vi "项名.vi"(8 "error in (no error)":errorcluster caption="错误输入（无错误）", 11 "LNK 输入":refnum<class "Hide Row.lvclass">) -> (0 "error out":errorcluster caption="错误输出", 3 "LNK 输出":refnum<class "Hide Row.lvclass">)   [LabVIEW 2016, in "Hide Row.lvclass"]
uses:
  Hide Row.lvclass
  Parent Class/Menu.lvclass
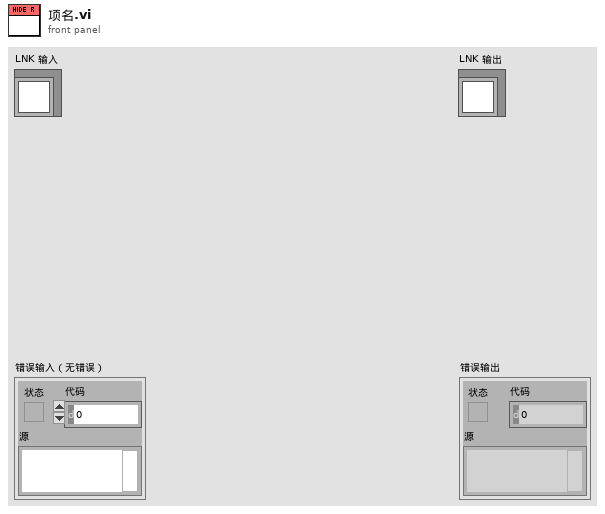
[diagram p1: front panel]
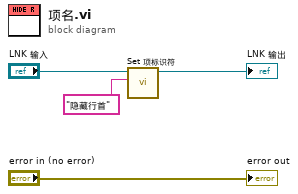
[diagram p0: block diagram]
diagram:
  n1 = call "Set 项标识符.vi"("项标识符"="隐藏行首", "LNK in"="LNK 输入") -> ("LNK out"=→"LNK 输出":refnum<class "Hide Row.lvclass">)  [unwired: 9 in]
  "error out" <- "error in (no error)"
